vi "Get database IP.vi"(8 "error in (no error)":errorcluster) -> (0 "error out":errorcluster, 1 "SQL Server Info":T2, 2 "value":string, 3 "Config file path":path)   [LabVIEW 2020]
uses:
  mysql_authentication.ctl
  <vilib>/Utility/config.llb/Read Key (String).vi
  <vilib>/Utility/config.llb/NI_LVConfig.lvlib
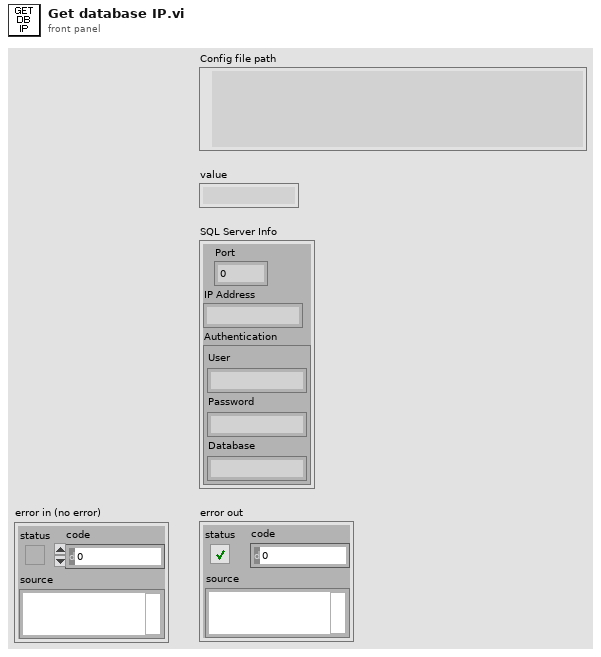
[diagram p1: front panel]
types:
  T1 = typedef "mysql_authentication.ctl" = cluster{"User":string, "Password":string, "Database":string}
  T2 = cluster{"Port":u16, "IP Address":string, "Authentication":T1}
  T3 = typedef "NI_LVConfig.lvlib/Config Data RefNum.ctl" = refnum<k1>
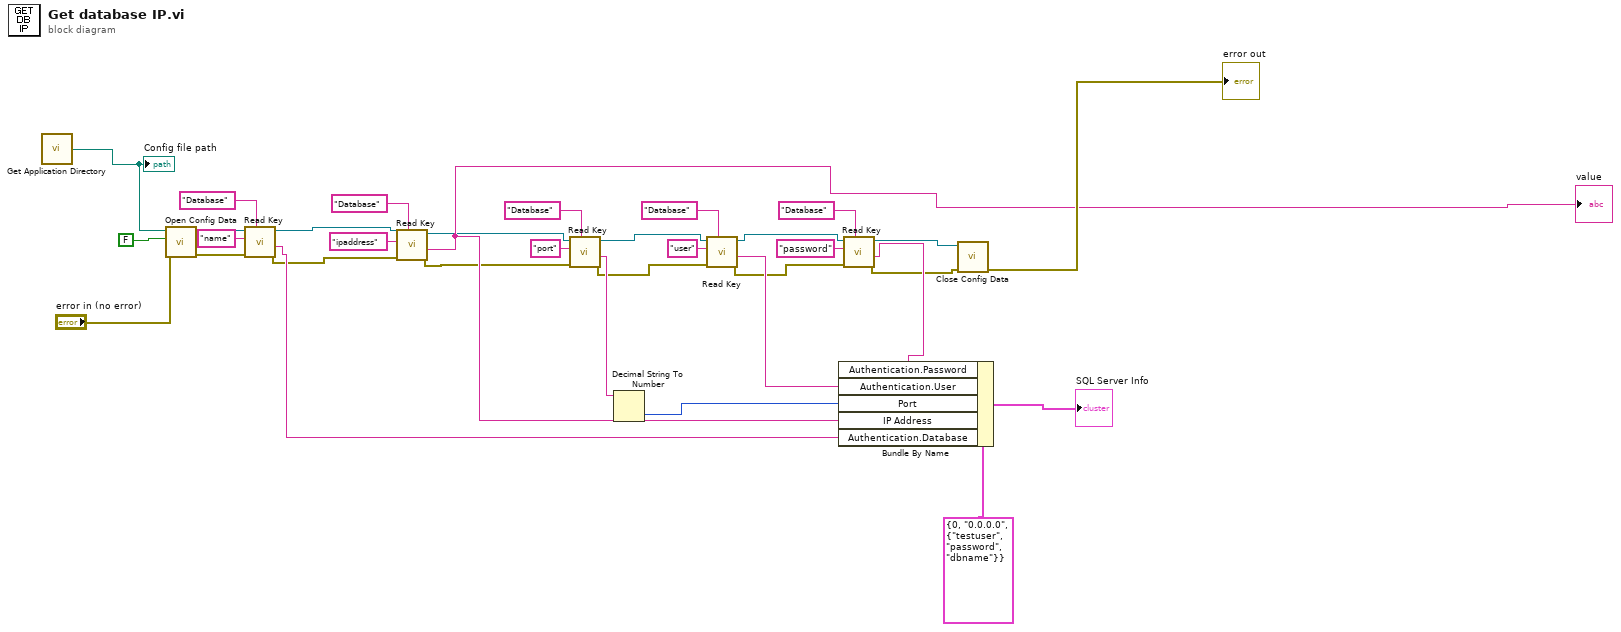
[diagram p0: block diagram]
diagram:
  n1 = call "Get Application Directory.vi"() -> ("Path to config file"=w1:path)  [unwired: 2 in]
  "Config file path" <- w1
  n2 = call <vilib>:"Open Config Data.vi"("error in (no error)"="error in (no error)", "create file if necessary (T)"=FALSE, "configuration file path"=w1) -> ("error out"=w24:errorcluster, "refnum"=w3:T3)  [unwired: 6 in, 1 out]
  n3 = call-poly <vilib>:"Read Key.vi"("section"="Database", "error in (no error)"=w24, "key"="name", "refnum"=w3) -> ("error out"=w23:errorcluster, "value"=w27:string, "refnum out"=w8:T3)  [unwired: 4 in, 1 out]
  n4 = call-poly <vilib>:"Read Key.vi"("section"="Database", "error in (no error)"=w23, "key"="ipaddress", "refnum"=w8) -> ("error out"=w22:errorcluster, "value"=w33:string, "refnum out"=w11:T3)  [unwired: 4 in, 1 out]
  "value" <- w33
  n5 = call-poly <vilib>:"Read Key.vi"("section"="Database", "error in (no error)"=w22, "key"="port", "refnum"=w11) -> ("error out"=w21:errorcluster, "value"=w28:string, "refnum out"=w16:T3)  [unwired: 4 in, 1 out]
  n6 = Decimal String To Number(string=w28) -> (number=w31:i32)  [unwired: 2 in, 1 out]
  n7 = call-poly <vilib>:"Read Key.vi"("section"="Database", "error in (no error)"=w21, "key"="user", "refnum"=w16) -> ("error out"=w20:errorcluster, "value"=w29:string, "refnum out"=w17:T3)  [unwired: 4 in, 1 out]
  n8 = call-poly <vilib>:"Read Key.vi"("section"="Database", "error in (no error)"=w20, "key"="password", "refnum"=w17) -> ("error out"=w19:errorcluster, "value"=w30:string, "refnum out"=w18:T3)  [unwired: 4 in, 1 out]
  n9 = Bundle By Name(cluster=T2 {"Port"=0, "IP Address"="0.0.0.0", "Authentication"={"User"="testuser", "Password"="password", "Database"="dbname"}} ("SQL Server Info"), "Authentication.Password"=w30, "Authentication.User"=w29, "Port"=w31, "IP Address"=w33, "Authentication.Database"=w27) -> (→"SQL Server Info":T2)
  n10 = call <vilib>:"Close Config Data.vi"("error in (no error)"=w19, "refnum"=w18) -> ("error out"=→"error out":errorcluster)  [unwired: 8 in, 1 out]
